vi "Register gRPC Server.vi"(8 "error in (no error)":errorcluster, 10 "gRPC ID":T1, 11 "CIFTemplateNode in":refnum<class "CIFCorePlugin.lvclass">) -> (0 "error out":errorcluster, 2 "gRPC ID Out":T1, 3 "CIFTemplateNode out":refnum<class "CIFCorePlugin.lvclass">)   [LabVIEW 2021, in "CIFCorePlugin.lvclass"]
uses:
  CIFCorePlugin.lvclass
  <vilib>/gRPC/LabVIEW gRPC Library/Shared/grpcId.ctl
  <vilib>/gRPC/LabVIEW gRPC Library/grpc-lvsupport-release.lvlib
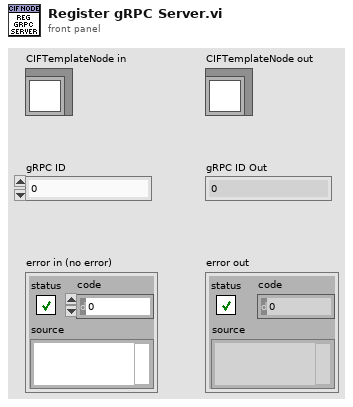
[diagram p1: front panel]
types:
  T1 = typedef "grpc-lvsupport-release.lvlib/grpcId.ctl" = u64
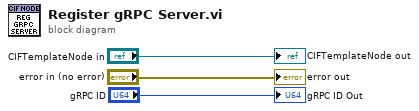
[diagram p0: block diagram]
diagram:
  "error out" <- "error in (no error)"
  "CIFTemplateNode out" <- "CIFTemplateNode in"
  "gRPC ID Out" <- "gRPC ID"
